vi "verify unique parameter in range.vi"(6 "lower limit":dbl, 7 "parameter name":string, 8 "error in (no error)":errorcluster, 9 "value":dbl, 10 "upper limit":dbl, 11 "Simulated_CCD_Camera in":refnum<class "Simulated Camera.lvclass">) -> (0 "error out":errorcluster, 3 "Simulated_CCD_Camera out":refnum<class "Simulated Camera.lvclass">)   [LabVIEW 2018, in "Simulated Camera.lvclass"]
uses:
  Simulated Camera.lvclass
  <vilib>/ErrorRing/Error Ring.xnode
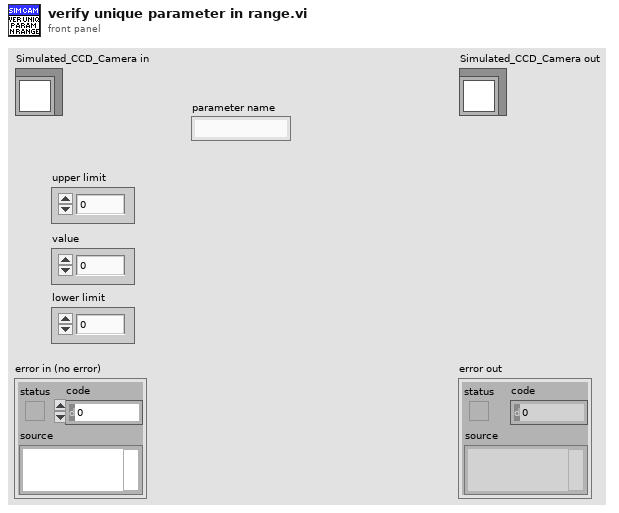
[diagram p1: front panel]
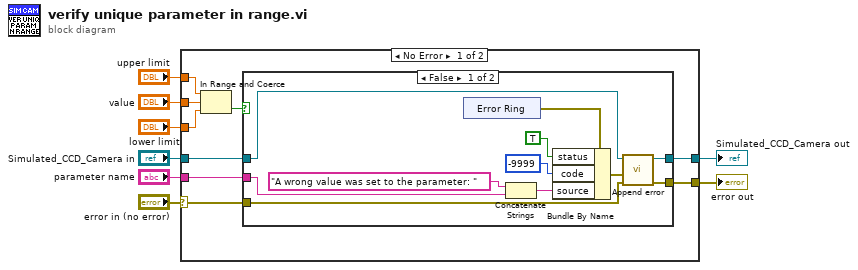
[diagram p0: block diagram]
diagram:
  n1 = case shown="No Error" "error in (no error)" {
    selector: "error in (no error)" -> [w10 w33]
    tunnel: [w9 w33] -> w7
    tunnel: [w17 w32] -> w6
    tunnel: "Simulated_CCD_Camera in" -> [w11 w32]
    tunnel: "lower limit" -> [w15 _]
    tunnel: "value" -> [w14 _]
    tunnel: "upper limit" -> [w13 _]
    tunnel: "parameter name" -> [w12 _]
    frame No Error {
      n2 = In Range and Coerce(upper limit=w13, x=w14, lower limit=w15) -> (In Range?=w16:bool)  [unwired: 1 out]
      n3 = case shown="False" w16 {
        tunnel: [w22 w31] -> w17
        tunnel: w11 -> [w21 w31]
        tunnel: w12 -> [w24 _]
        tunnel: w10 -> [w19 w30]
        tunnel: [w18 w30] -> w9
        frame False {
          n4 = xnode "Error Ring"() -> ("error out"=w28:errorcluster)
          n5 = Concatenate Strings("A wrong value was set to the parameter: " ("string"), w24) -> (w27:string)
          n6 = Bundle By Name(cluster=w28, "status"=TRUE, "code"=-9999, "source"=w27) -> (w20:errorcluster)
          n7 = call "Append error.vi"("error in (no error)"=w19, "error"=w20, "Simulated_CCD_Camera in"=w21) -> ("error out"=w18:errorcluster, "Simulated_CCD_Camera out"=w22:refnum<class "Simulated Camera.lvclass">)  [unwired: 7 in]
        }
        frame True {
        }
      }
    }
    frame Error {
    }
  }
  "error out" <- w7
  "Simulated_CCD_Camera out" <- w6
